vi "Untitled 1.vi"() -> ()   [LabVIEW 2016]
uses:
  <vilib>/Analysis/Matrix/Numeric/Conversions/Array To Matrix - RA2.vi
  <vilib>/imath/engines/lvmath2/RunTimeEngine/Managers/WorkSpace/UID Generator.vi
  <vilib>/Analysis/Matrix/Numeric/Conversions/Matrix To Array - RM.vi
  <vilib>/imath/engines/lvmath2/RunTimeEngine/BuiltInFunctions/round/NIMS_round(DBL-S).vi
  <vilib>/imath/engines/lvmath2/RunTimeEngine/RunTimeType/NIMS_RunTimeType_From StrictType (excl LVString).vi
  <instcachedir>/0/NIMS_RunTimeType_From StrictType (excl LVString)_BBF44FB49F834B71AF7A14CCEDF8BECD.lvgen/NIMS_RunTimeType_From StrictType (excl LVString)_BBF44FB49F834B71AF7A14CCEDF8BECD_000.vi
  <vilib>/imath/engines/lvmath2/RunTimeEngine/LocalVariableDefStatement/MC_LocalVariableDefStatement_Display.vi
  <vilib>/imath/engines/lvmath2/RunTimeEngine/BuiltInFunctions/rotate90/NIMS_rotate90.vi
  <instcachedir>/0/NIMS_rotate90_7DC1660D109944E092D2EB6E3185A1B6.lvgen/NIMS_rotate90_7DC1660D109944E092D2EB6E3185A1B6_004.vi
  <vilib>/imath/engines/lvmath2/RunTimeEngine/Managers/SymbolTable/Clear UID.vi
  <vilib>/imath/engines/lvmath2/RunTimeEngine/NodeEndStatement/NIMS_NodeEndStatement_Output.vi
  <instcachedir>/0/NIMS_NodeEndStatement_Output_53EC0D466D134D7ABD903AC30B43404B.lvgen/NIMS_NodeEndStatement_Output_53EC0D466D134D7ABD903AC30B43404B_002.vi
  <vilib>/imath/engines/lvmath2/RunTimeEngine/ErrorHandling/NIMS_Finalize Error.vi
  <vilib>/picture/picture.llb/Draw True-Color Pixmap.vi
  <vilib>/Analysis/Matrix/NI_Matrix.lvlib
  <vilib>/imath/engines/lvmath2/RunTimeEngine/Managers/SymbolTable/NIMS_WorkSpace.lvlib
panel:
  out "output cluster":T1
  in  "Meter":dbl(knob) scale=-360.0..360.0
  out "number":u32
  out "new picture 2":picture
  in  "y":dbl(slide) scale=-500.0..500.0
  in  "x":dbl(slide) scale=-500.0..500.0
  in  "Enum":enum16{"translacion", "giro"}(ring)
  out "new picture":picture
  in  "File Path Control":path
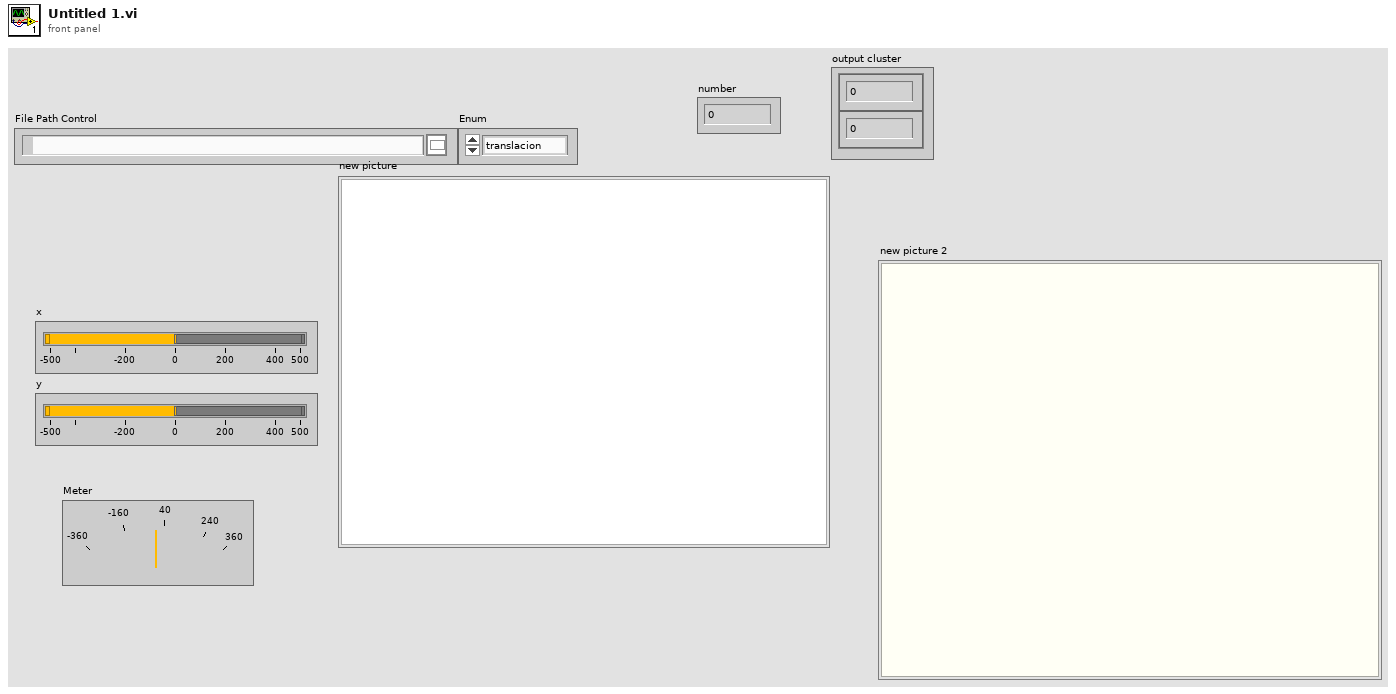
[diagram p1: front panel]
types:
  T1 = cluster{"Numeric Control":dbl, "Numeric Control":dbl}
  T2 = typedef "imagedata.ctl" = cluster{"image type":i32, "image depth":i32, "image":u8[], "mask":u8[], "colors":u32[], "Rectangle":cluster{"left":i16, "top":i16, "right":i16, "bottom":i16}}
  T3 = typedef "NI_Matrix.lvlib/RealMatrix.ctl" = dbl[][]
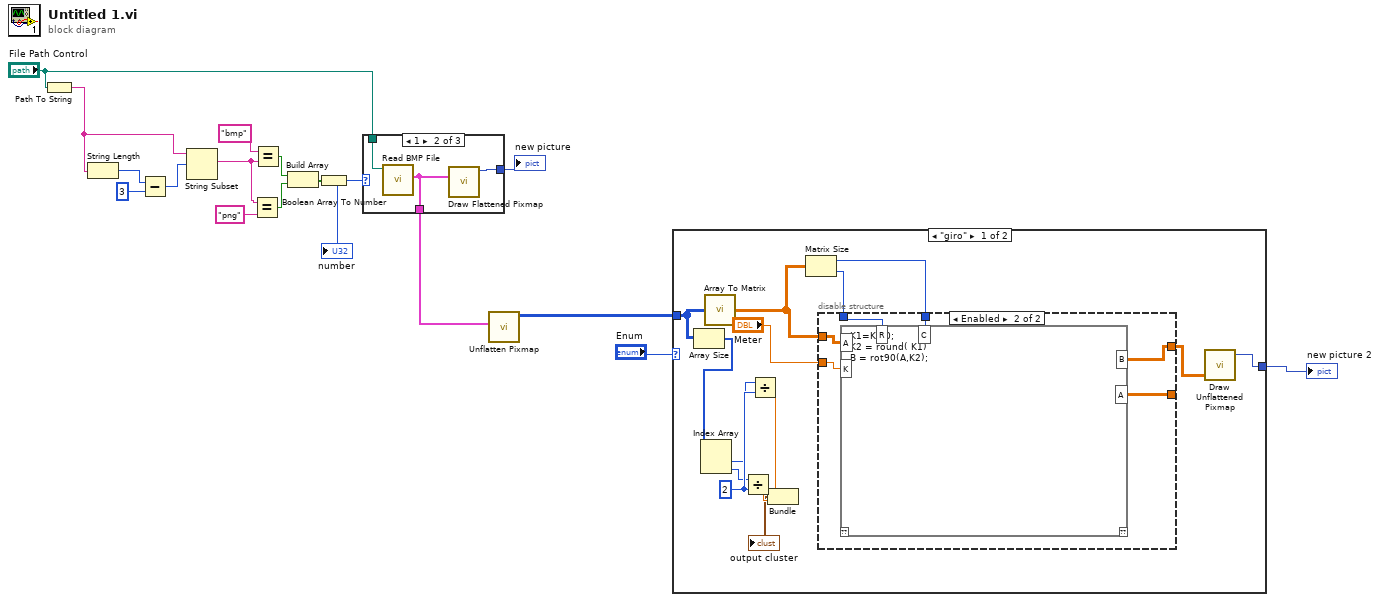
[diagram p0: block diagram]
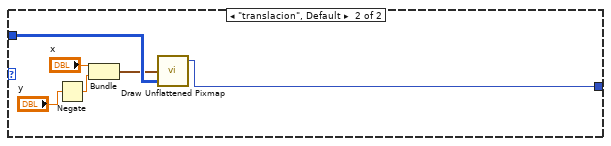
[diagram p3: hidden frame]
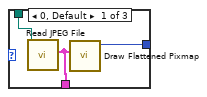
[diagram p4: hidden frame]
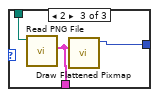
[diagram p5: hidden frame]
diagram:
  n1 = Path To String(path="File Path Control") -> (string=w14:string)
  n2 = String Length(string=w14) -> (length=w17:i32)
  n3 = Subtract(x=w17, y=3) -> (x-y=w15:i32)
  n4 = String Subset(string=w14, offset (0)=w15) -> (substring=w11:string)  [unwired: 1 in]
  n5 = Equal?(x=w11, y="png" ("x")) -> (x = y?=w8:bool)
  n6 = Equal?(x="bmp", y=w11) -> (x = y?=w7:bool)
  n7 = Build Array(w7, w8) -> (w9:bool[])
  n8 = Boolean Array To Number(Boolean array=w9) -> (number=w10:u32)
  "number" <- w10
  n9 = case shown="1" w10 {
    tunnel: [w20 w23 w25] -> w2
    tunnel: "File Path Control" -> [w19 w22 w26]
    tunnel: [w18 w21 w24] -> w1
    frame 0, Default {
      n10 = call <vilib>:"Read JPEG File.vi"("path to JPEG file"=w19) -> ("image data"=w18:T2)  [unwired: 8 in, 2 out]
      n11 = call <vilib>:"Draw Flattened Pixmap.vi"("image data"=w18) -> ("new picture"=w20:picture)  [unwired: 8 in]
    }
    frame 1 {
      n12 = call <vilib>:"Read BMP File.vi"("path to BMP file"=w22) -> ("image data"=w21:T2)  [unwired: 8 in, 2 out]
      n13 = call <vilib>:"Draw Flattened Pixmap.vi"("image data"=w21) -> ("new picture"=w23:picture)  [unwired: 8 in]
    }
    frame 2 {
      n14 = call <vilib>:"Read PNG File.vi"("path to PNG file"=w26) -> ("image data"=w24:T2)  [unwired: 8 in, 2 out]
      n15 = call <vilib>:"Draw Flattened Pixmap.vi"("image data"=w24) -> ("new picture"=w25:picture)  [unwired: 8 in]
    }
  }
  "new picture" <- w2
  n16 = call <vilib>:"Unflatten Pixmap.vi"("image data"=w1) -> ("24-bit pixmap"=w3:u32[][])  [unwired: 4 in, 6 out]
  n17 = case shown="\"giro\"" "Enum" {
    tunnel: [w29 w109] -> w5
    tunnel: w3 -> [w34 w108]
    frame "giro" {
      w40 = 2 ("y")
      n18 = Array Size(array=w34) -> (size(s)=w37:i32[])
      n19 = Index Array(array=w37) -> (element #1=w36:i32, element #2=w35:i32)  [unwired: 2 in]
      n20 = call-poly <vilib>:"Array To Matrix.vi"("Real 2D Array"=w34) -> ("Real Matrix"=w32:T3)
      n21 = Divide(x=w35, y=w40) -> (x/y=w38:dbl)
      n22 = Divide(x=w36, y=w40) -> (x/y=w39:dbl)
      n23 = Bundle(w39, w38) -> (→"output cluster":cluster{dbl, dbl})  [unwired: 1 in]
      n24 = Matrix Size(0:w32) -> (1:w31:i32, 2:w30:i32)
      n25 = disable-structure shown="Enabled" {
        disable-tunnel: "Meter" -> [_ w46]
        disable-tunnel: w32 -> [_ w45]
        disable-tunnel: w31 -> [_ w43]
        disable-tunnel: w30 -> [_ w44]
        disable-tunnel: [_ w42] -> w27
        disable-tunnel: [_ w41] -> _
        frame Disabled {
        }
        frame Enabled {
          n26 = mathscript code="K1=K/90;\nK2 = round( K1)\nB = rot90(A,K2);"("A"=w45, "K"=w46, "R"=w44, "C"=w43) -> ("B"=w42:dbl[][], "A"=w41:dbl[][])  [unwired: 1 in, 1 out]
        }
      }
      n27 = call-poly <vilib>:"Draw Unflattened Pixmap.vi"("data (RGB format)"=w27) -> ("new picture"=w29:picture)  [unwired: 8 in]
    }
    frame "translacion", Default {
      n28 = Negate(x="y") -> (-x=w107:dbl)
      n29 = Bundle("x"="x", w107) -> (w104:cluster{"x":dbl, dbl})  [unwired: 1 in]
      n30 = call-poly <vilib>:"Draw Unflattened Pixmap.vi"("top left point(0, 0)"=w104, "data (RGB format)"=w108) -> ("new picture"=w109:picture)  [unwired: 7 in]
    }
  }
  "new picture 2" <- w5
